vi "motor_lv.vi"(4 "error in":errorcluster, 6 "Request data":variant, 7 "Request":string) -> (0 "error out":errorcluster, 2 "Response data":variant)   [LabVIEW 2018]
panel:
  in  "Python session":refnum<k35>
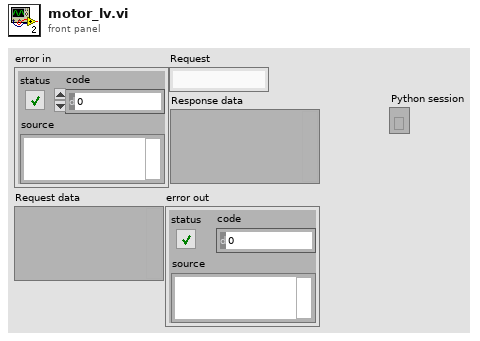
[diagram p1: front panel]
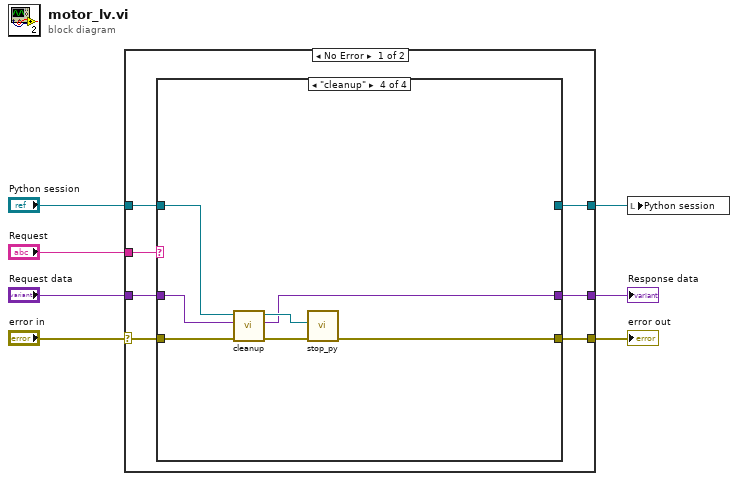
[diagram p0: block diagram]
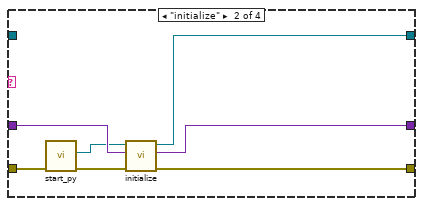
[diagram p3: hidden frame]
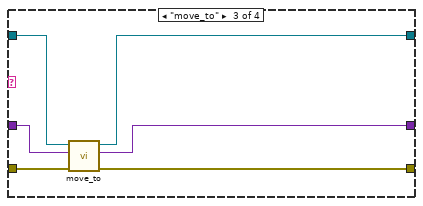
[diagram p4: hidden frame]
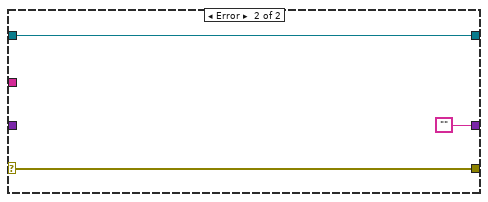
[diagram p5: hidden frame]
diagram:
  n1 = case shown="No Error" "error in" {
    selector: "error in" -> [w13 w40]
    tunnel: [w11 w40] -> w6
    tunnel: "Request" -> [w14 _]
    tunnel: "Request data" -> [w12 _]
    tunnel: [w10 ""] -> w3
    tunnel: "Python session" -> [w9 w38]
    tunnel: [w8 w38] -> w2
    frame No Error {
      n2 = case shown="\"cleanup\"" w14 {
        tunnel: w13 -> [w16 w24 w30 w36]
        tunnel: w12 -> [w17 w22 w29 w34]
        tunnel: [w16 w18 w25 w37] -> w11
        tunnel: [w17 w20 w26 w31] -> w10
        tunnel: w9 -> [w15 _ w28 w33]
        tunnel: [w15 w19 w27 _] -> w8
        frame "", Default {
        }
        frame "initialize" {
          n3 = call "start_py.vi"("error in"=w24) -> ("error out"=w23:errorcluster, "Python session"=w21:refnum<k35>)  [unwired: 5 in]
          n4 = call "initialize.vi"("error in (no error)"=w23, "Request data"=w22, "Python session in"=w21) -> ("error out"=w18:errorcluster, "Response data"=w20:variant, "Python session out"=w19:refnum<k35>)  [unwired: 2 in]
        }
        frame "move_to" {
          n5 = call "move_to.vi"("error in (no error)"=w30, "Request data"=w29, "Python session in"=w28) -> ("error out"=w25:errorcluster, "Response data"=w26:variant, "Python session out"=w27:refnum<k35>)  [unwired: 2 in]
        }
        frame "cleanup" {
          n6 = call "cleanup.vi"("error in (no error)"=w36, "Request data"=w34, "Python session in"=w33) -> ("error out"=w35:errorcluster, "Response data"=w31:variant, "Python session out"=w32:refnum<k35>)  [unwired: 2 in]
          n7 = call "stop_py.vi"("error in"=w35, "Python session"=w32) -> ("error out"=w37:errorcluster)  [unwired: 5 in]
        }
      }
    }
    frame Error {
    }
  }
  "Response data" <- w3
  "error out" <- w6
  n8 = local write "Python session"(w2) -> ()
